vi "subFD_Filter Coef.vi"(10 "Coef b (v)":dbl[](array[numeric]) format="%#_10g", 11 "Coef a (k)":dbl[](array[numeric]) format="%#_10g") -> (3 "Coefficients Report":string)   [LabVIEW 2023]
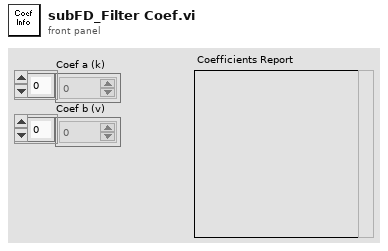
[diagram p1: front panel]
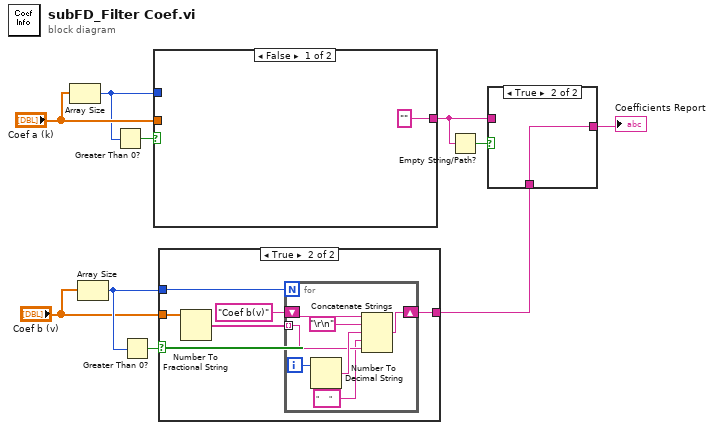
[diagram p0: block diagram]
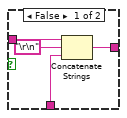
[diagram p2: hidden frame]
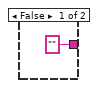
[diagram p3: hidden frame]
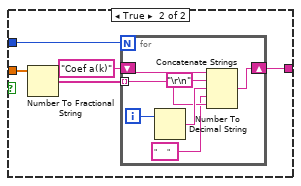
[diagram p4: hidden frame]
diagram:
  n1 = Array Size(array="Coef a (k)") -> (size(s)=w8:i32)
  n2 = Array Size(array="Coef b (v)") -> (size(s)=w6:i32)
  n3 = Greater Than 0?(x=w8) -> (x > 0?=w9:bool)
  n4 = Greater Than 0?(x=w6) -> (x > 0?=w7:bool)
  n5 = case shown="False" w9 {
    tunnel: "Coef a (k)" -> [_ w15]
    tunnel: w8 -> [_ w13]
    tunnel: ["" ("Coefficients Report") w12] -> w2
    frame False {
    }
    frame True {
      n6 = Number To Fractional String(number=w15) -> (F-format string=w14:string[])  [unwired: 3 out]
      n7 = for {
        N: w13 -> [_]
        shift-right: [w23] -> w12
        shift-left: "Coef a(k)" ("Coefficients Report") -> [w22]
        tunnel: w14 -> [w18] mode=indexing
        i -> [w20]
        n8 = Number To Decimal String(number=w20) -> (decimal integer string=w19:string)  [unwired: 1 out]
        n9 = Concatenate Strings(w22, "\r\n", w19, "     ", w18) -> (w23:string)
      }
    }
  }
  n10 = case shown="True" w7 {
    tunnel: w6 -> [_ w27]
    tunnel: "Coef b (v)" -> [_ w26]
    tunnel: ["" ("Coefficients Report") w25] -> w4
    frame False {
    }
    frame True {
      n11 = Number To Fractional String(number=w26) -> (F-format string=w29:string[])  [unwired: 3 out]
      n12 = for {
        N: w27 -> [_]
        shift-right: [w36] -> w25
        shift-left: "Coef b(v)" ("Coefficients Report") -> [w35]
        tunnel: w29 -> [w31] mode=indexing
        i -> [w33]
        n13 = Number To Decimal String(number=w33) -> (decimal integer string=w32:string)  [unwired: 1 out]
        n14 = Concatenate Strings(w35, "\r\n", w32, "     ", w31) -> (w36:string)
      }
    }
  }
  n15 = Empty String/Path?(string/path=w2) -> (empty?=w1:bool)
  n16 = case shown="True" w1 {
    tunnel: w4 -> [w39 w41]
    tunnel: [w38 w41] -> w3
    tunnel: w2 -> [w37 _]
    frame False {
      n17 = Concatenate Strings(w37, "\r\n", w39) -> (w38:string)
    }
    frame True {
    }
  }
  "Coefficients Report" <- w3
